vi "q_update_add_q.vi"(0 "Q1_orig":fxp<+/-,32,16>, 1 "Q2_orig":fxp<+/-,32,16>, 2 "Q3_orig":fxp<+/-,32,16>, 3 "Q4_orig":fxp<+/-,32,16>, 4 "q1_valid":bool, 5 "Q1_temp":fxp<+/-,32,16>, 6 "q2_valid":bool, 7 "Q2_temp":fxp<+/-,32,16>, 8 "q3_valid":bool, 9 "Q3_temp":fxp<+/-,32,16>, 10 "q4_valid":bool, 11 "Q4_temp":fxp<+/-,32,16>) -> (12 "Q1_update":fxp<+/-,32,16>, 13 "q4_ready":bool, 14 "q1_ready":bool, 15 "Q2_update":fxp<+/-,32,16>, 16 "q2_ready":bool, 17 "Q3_update":fxp<+/-,32,16>, 18 "q3_ready":bool, 19 "Q4_update":fxp<+/-,32,16>)   [LabVIEW 2020]
uses:
  <vilib>/rvi/FXPMathLib/FxpAdd/XNode/nifxpmath_Add.xnode
  <vilib>/rvi/FXPMathLib/sim/FxpSim.dll
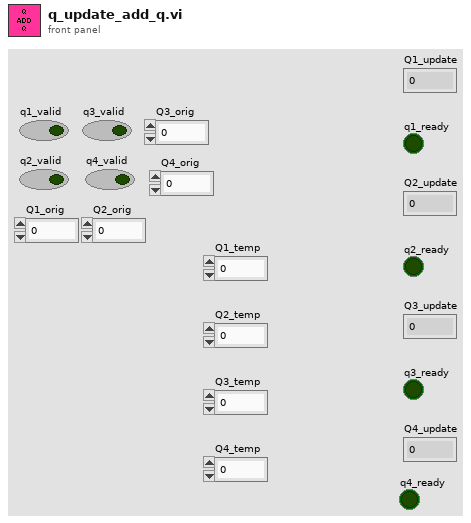
[diagram p1: front panel]
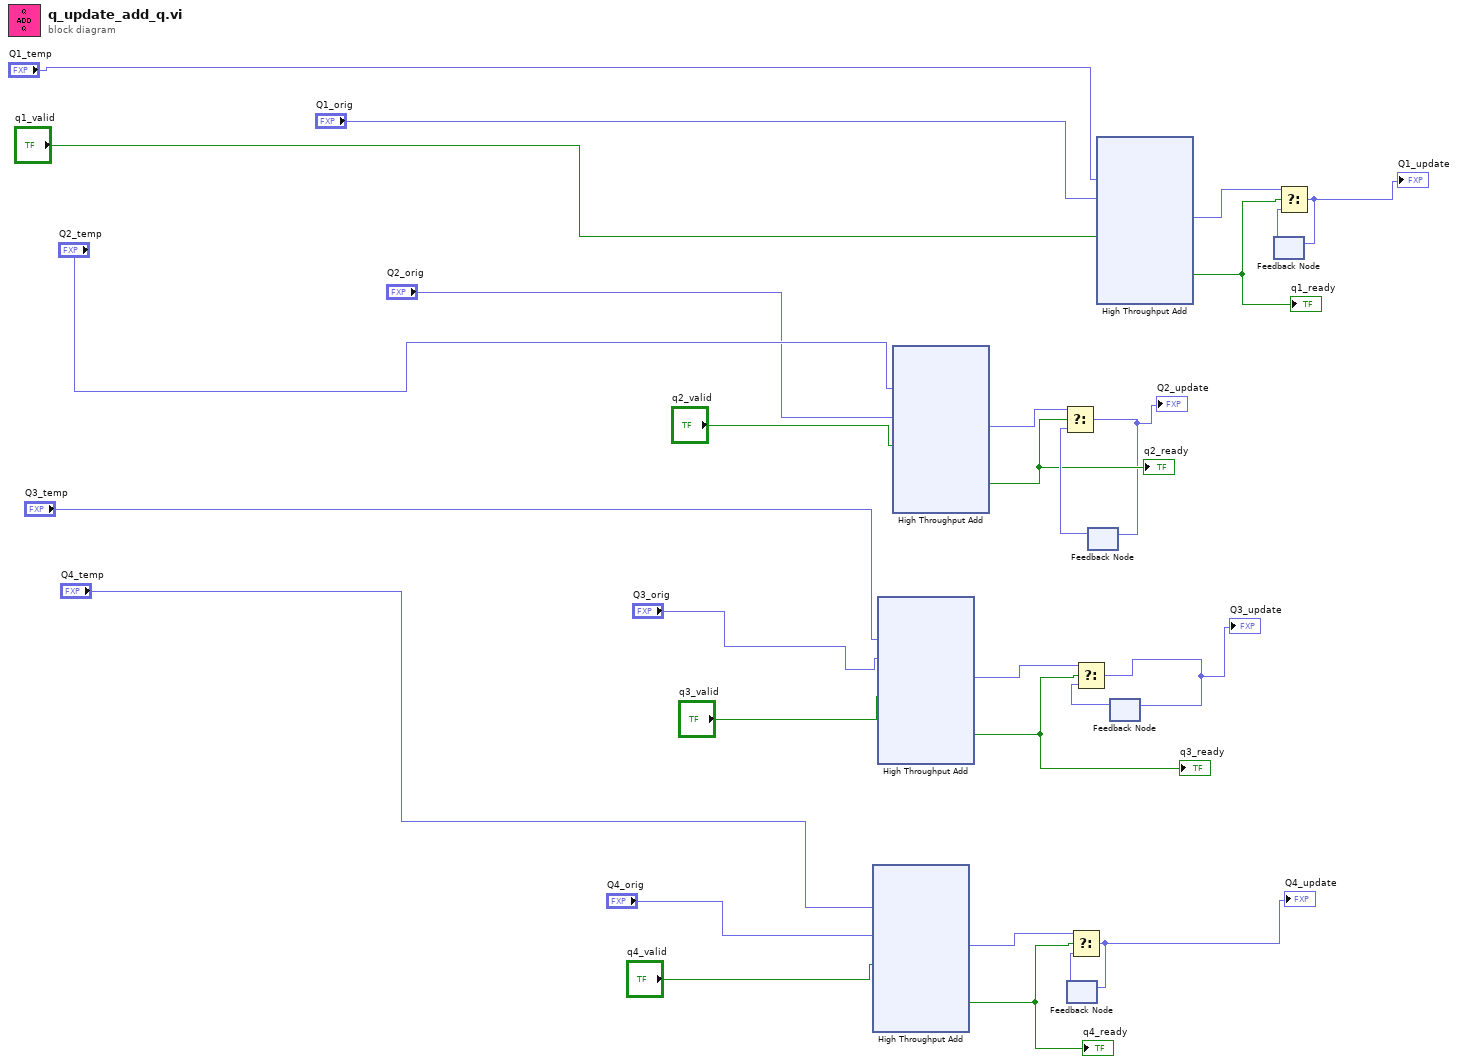
[diagram p0: block diagram]
diagram:
  n1 = xnode "High Throughput Add"("x"="Q4_temp", "y"="Q4_orig", "input valid"="q4_valid") -> ("x+y"=w26:fxp<+/-,32,16>, "output valid"=w25:bool)  [unwired: 1 in, 1 out]
  "q4_ready" <- w25
  n2 = xnode "High Throughput Add"("x"="Q3_temp", "y"="Q3_orig", "input valid"="q3_valid") -> ("x+y"=w23:fxp<+/-,32,16>, "output valid"=w22:bool)  [unwired: 1 in, 1 out]
  "q3_ready" <- w22
  n3 = xnode "High Throughput Add"("x"="Q2_temp", "y"="Q2_orig", "input valid"="q2_valid") -> ("x+y"=w20:fxp<+/-,32,16>, "output valid"=w19:bool)  [unwired: 1 in, 1 out]
  "q2_ready" <- w19
  n4 = feedback #1() -> (w27:fxp<+/-,32,16>)  [unwired: 1 in]
  n5 = Select(t=w26, s=w25, f=w27) -> (s? t:f=w1:fxp<+/-,32,16>)
  "Q4_update" <- w1
  n6 = feedback-in #1(w1) -> ()
  n7 = feedback #2() -> (w21:fxp<+/-,32,16>)  [unwired: 1 in]
  n8 = Select(t=w20, s=w19, f=w21) -> (s? t:f=w3:fxp<+/-,32,16>)
  "Q2_update" <- w3
  n9 = feedback-in #2(w3) -> ()
  n10 = xnode "High Throughput Add"("x"="Q1_temp", "y"="Q1_orig", "input valid"="q1_valid") -> ("x+y"=w17:fxp<+/-,32,16>, "output valid"=w16:bool)  [unwired: 1 in, 1 out]
  "q1_ready" <- w16
  n11 = feedback #3() -> (w24:fxp<+/-,32,16>)  [unwired: 1 in]
  n12 = Select(t=w23, s=w22, f=w24) -> (s? t:f=w2:fxp<+/-,32,16>)
  "Q3_update" <- w2
  n13 = feedback-in #3(w2) -> ()
  n14 = feedback #4() -> (w18:fxp<+/-,32,16>)  [unwired: 1 in]
  n15 = Select(t=w17, s=w16, f=w18) -> (s? t:f=w4:fxp<+/-,32,16>)
  "Q1_update" <- w4
  n16 = feedback-in #4(w4) -> ()
